vi "Realtime_interaction VI.vi"() -> ()   [LabVIEW 2020]
uses:
  <vilib>/FPGAPlugInAG/cRIO-9054/niLvFpga_Open_cRIO-9054.vi
  <vilib>/rvi/interface/common/dynamic/niFpgaDynamicAddResources.vi
  <vilib>/Utility/error.llb/Error Cluster From Error Code.vi
  <vilib>/rvi/errors/niLvFpgaAdjustHostInterfaceError.vi
  <vilib>/FPGAPlugInAG/Dynamic/niLvFpga_Close_Dynamic.vi
  <vilib>/rvi/interface/nirviOpenFPGA/nirviOpenFPGA.xnode
  FPGA Bitfiles/ver0.1_FPGATarget_FPGAcontrolledVI_cWk4O34ijhk.lvbitx
  FPGA_controlled VI.vi
  <vilib>/rvi/interface/nirviReadWriteControl/nirviReadWriteControl.xnode
  <vilib>/rvi/interface/nirviCloseFPGA/nirviCloseFPGA.xnode
  NiFpgaLv.dll
  <vilib>/rvi/interface/Simulation/niFpgaSimulationCallBeginRW.vi
panel:
  out "Mod1/AI0":fxp<+/-,26,5>
  in  "stop":bool
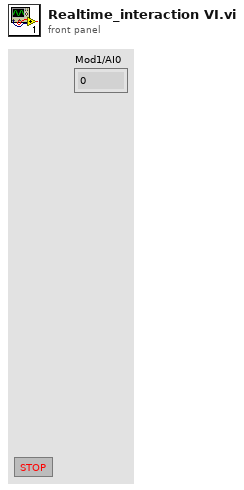
[diagram p1: front panel]
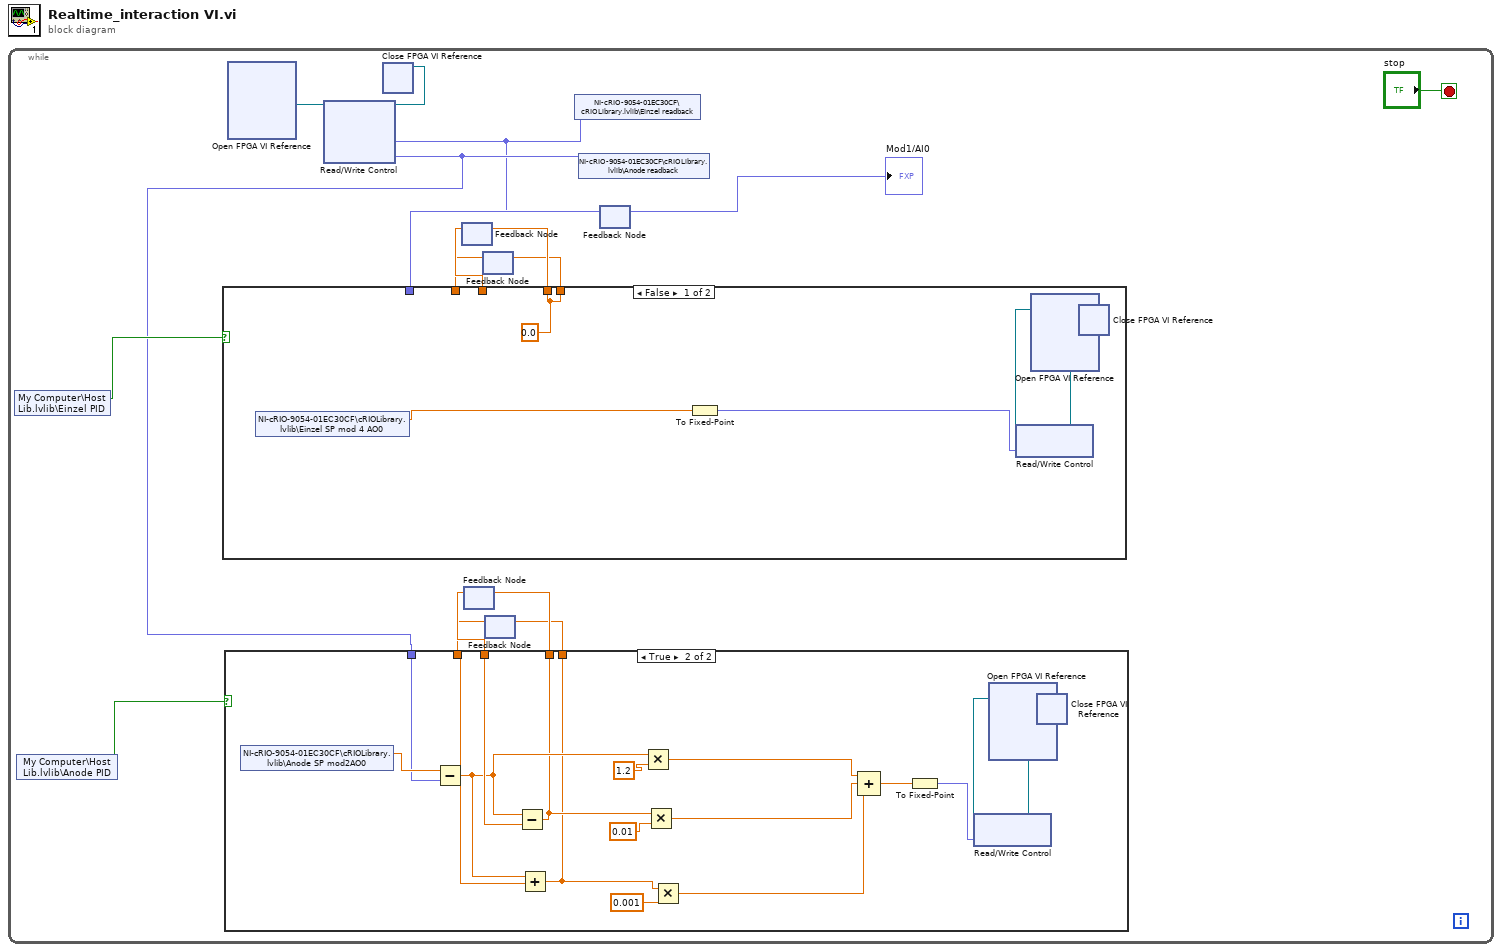
[diagram p0: block diagram]
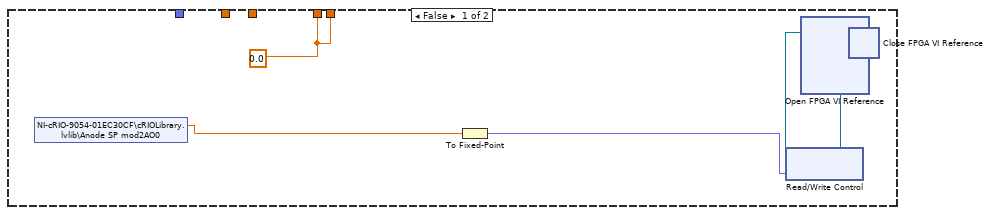
[diagram p2: hidden frame]
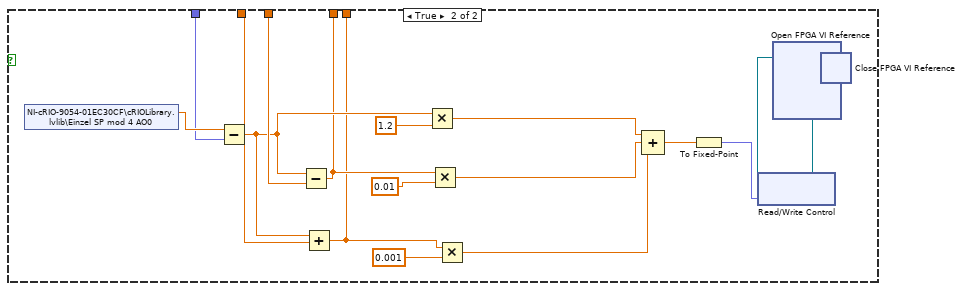
[diagram p3: hidden frame]
diagram:
  n1 = while {
    stop <- "stop" stop-if-true
    n2 = shared-variable "My Computer\\Host Lib.lvlib\\Einzel PID"() -> (w13:bool)  [unwired: 1 in, 1 out]
    n3 = shared-variable "My Computer\\Host Lib.lvlib\\Anode PID"() -> (w7:bool)  [unwired: 1 in, 1 out]
    n4 = xnode "Open FPGA VI Reference"() -> ("FPGA VI Reference Out"=w15:refnum<k20>)  [unwired: 2 in, 1 out]
    n5 = xnode "Read/Write Control"("FPGA VI Reference In"=w15) -> ("FPGA VI Reference Out"=w14:refnum<k20>, "Mod1/AI0"=w1:fxp<+/-,26,5>, "Mod1/AI2"=w2:fxp<+/-,26,5>)  [unwired: 2 in, 1 out]
    n6 = xnode "Close FPGA VI Reference"("FPGA VI Reference In"=w14) -> ()  [unwired: 1 in, 1 out]
    n7 = feedback #1() -> (w10:dbl)  [unwired: 1 in]
    n8 = feedback #2() -> (w5:dbl)  [unwired: 1 in]
    n9 = feedback #3() -> (w8:dbl)  [unwired: 1 in]
    n10 = feedback #4() -> (w3:dbl)  [unwired: 1 in]
    n11 = case shown="True" w7 {
      tunnel: w2 -> [_ w37]
      tunnel: w5 -> [_ w36]
      tunnel: [w17 w33] -> w6
      tunnel: [w17 w31] -> w4
      tunnel: w3 -> [_ w34]
      frame False {
        w17 = 0.0
        n12 = shared-variable "NI-cRIO-9054-01EC30CF\\cRIOLibrary.lvlib\\Anode SP mod2AO0"() -> (w18:dbl)  [unwired: 1 in, 1 out]
        n13 = To Fixed-Point(number=w18) -> (fixed-point=w19:fxp<+/-,20,5>)  [unwired: 1 in]
        n14 = xnode "Open FPGA VI Reference"() -> ("FPGA VI Reference Out"=w20:refnum<k20>)  [unwired: 2 in, 1 out]
        n15 = xnode "Read/Write Control"("FPGA VI Reference In"=w20, "Mod2/AO0"=w19) -> ("FPGA VI Reference Out"=w21:refnum<k20>)  [unwired: 1 in, 1 out]
        n16 = xnode "Close FPGA VI Reference"("FPGA VI Reference In"=w21) -> ()  [unwired: 1 in, 1 out]
      }
      frame True {
        n17 = shared-variable "NI-cRIO-9054-01EC30CF\\cRIOLibrary.lvlib\\Anode SP mod2AO0"() -> (w38:dbl)  [unwired: 1 in, 1 out]
        n18 = Subtract(x=w38, y=w37) -> (x-y=w35:dbl)
        n19 = Subtract(x=w35, y=w36) -> (x-y=w33:dbl)
        n20 = Add(x=w35, y=w34) -> (x+y=w31:dbl)
        n21 = Multiply(x=w35, y=1.2) -> (x*y=w30:dbl)
        n22 = Multiply(x=w33, y=0.01) -> (x*y=w32:dbl)
        n23 = Multiply(x=w31, y=0.001) -> (x*y=w29:dbl)
        n24 = Compound Arithmetic op=ADD(w30, w32, w29) -> (w25:dbl)
        n25 = To Fixed-Point(number=w25) -> (fixed-point=w26:fxp<+/-,20,5>)  [unwired: 1 in]
        n26 = xnode "Open FPGA VI Reference"() -> ("FPGA VI Reference Out"=w28:refnum<k20>)  [unwired: 2 in, 1 out]
        n27 = xnode "Read/Write Control"("FPGA VI Reference In"=w28, "Mod2/AO0"=w26) -> ("FPGA VI Reference Out"=w27:refnum<k20>)  [unwired: 1 in, 1 out]
        n28 = xnode "Close FPGA VI Reference"("FPGA VI Reference In"=w27) -> ()  [unwired: 1 in, 1 out]
      }
    }
    n29 = feedback-in #2(w6) -> ()
    n30 = feedback-in #4(w4) -> ()
    n31 = shared-variable "NI-cRIO-9054-01EC30CF\\cRIOLibrary.lvlib\\Einzel readback"(w1) -> ()  [unwired: 1 in, 1 out]
    n32 = shared-variable "NI-cRIO-9054-01EC30CF\\cRIOLibrary.lvlib\\Anode readback"(w2) -> ()  [unwired: 1 in, 1 out]
    n33 = feedback-in #5(w1) -> ()
    n34 = feedback #5() -> (w12:fxp<+/-,26,5>)  [unwired: 1 in]
    "Mod1/AI0" <- w12
    n35 = case shown="False" w13 {
      tunnel: w12 -> [_ w59]
      tunnel: w10 -> [_ w58]
      tunnel: [w40 w55] -> w11
      tunnel: [w40 w53] -> w9
      tunnel: w8 -> [_ w56]
      frame False {
        w40 = 0.0
        n36 = shared-variable "NI-cRIO-9054-01EC30CF\\cRIOLibrary.lvlib\\Einzel SP mod 4 AO0"() -> (w39:dbl)  [unwired: 1 in, 1 out]
        n37 = To Fixed-Point(number=w39) -> (fixed-point=w41:fxp<+/-,20,5>)  [unwired: 1 in]
        n38 = xnode "Open FPGA VI Reference"() -> ("FPGA VI Reference Out"=w42:refnum<k20>)  [unwired: 2 in, 1 out]
        n39 = xnode "Read/Write Control"("FPGA VI Reference In"=w42, "Mod4/AO0"=w41) -> ("FPGA VI Reference Out"=w43:refnum<k20>)  [unwired: 1 in, 1 out]
        n40 = xnode "Close FPGA VI Reference"("FPGA VI Reference In"=w43) -> ()  [unwired: 1 in, 1 out]
      }
      frame True {
        n41 = shared-variable "NI-cRIO-9054-01EC30CF\\cRIOLibrary.lvlib\\Einzel SP mod 4 AO0"() -> (w60:dbl)  [unwired: 1 in, 1 out]
        n42 = Subtract(x=w60, y=w59) -> (x-y=w57:dbl)
        n43 = Subtract(x=w57, y=w58) -> (x-y=w55:dbl)
        n44 = Add(x=w57, y=w56) -> (x+y=w53:dbl)
        n45 = Multiply(x=w57, y=1.2) -> (x*y=w52:dbl)
        n46 = Multiply(x=w55, y=0.01) -> (x*y=w54:dbl)
        n47 = Multiply(x=w53, y=0.001) -> (x*y=w51:dbl)
        n48 = Compound Arithmetic op=ADD(w52, w54, w51) -> (w47:dbl)
        n49 = To Fixed-Point(number=w47) -> (fixed-point=w48:fxp<+/-,20,5>)  [unwired: 1 in]
        n50 = xnode "Open FPGA VI Reference"() -> ("FPGA VI Reference Out"=w50:refnum<k20>)  [unwired: 2 in, 1 out]
        n51 = xnode "Read/Write Control"("FPGA VI Reference In"=w50, "Mod4/AO0"=w48) -> ("FPGA VI Reference Out"=w49:refnum<k20>)  [unwired: 1 in, 1 out]
        n52 = xnode "Close FPGA VI Reference"("FPGA VI Reference In"=w49) -> ()  [unwired: 1 in, 1 out]
      }
    }
    n53 = feedback-in #1(w11) -> ()
    n54 = feedback-in #3(w9) -> ()
  }
